vi "Stanford Research 830 Expand Offset and Output Channel.vi"() -> ()   [LabVIEW 2019]
doc: "This example shows how to configure all the channel-related parameters of the instrument to get the desired output value."
uses:
  Stanford Research 830.lvlib
panel:
  in  "Offset/Expand Parameter (1: X)":u16(ring)=1 items=["X"=1, "Y"=2, "R"=3]
  in  "Expand (0: x1)":u16(ring) items=["x1", "x10", "x100"]
  in  "Channel 1 Display With Ratio (0: None)":u16(ring) items=["None", "Aux In 1", "Aux In 2"]
  in  "Channel 1 Display (0: X)":u16(ring) items=["X", "R", "X Noise", "Aux In 1", "Aux In 2"]
  in  "Manual Offset (40)":dbl=40.0
  in  "Auto Offset (F: Disable)":bool
  in  "VISA resource name":refnum<visa-resource-name>
  # "(c) 2006 National Instruments.  ALL RIGHTS RESERVED."
  # "Offset/Expand Configuration"
  # "Channel Display Configuration"
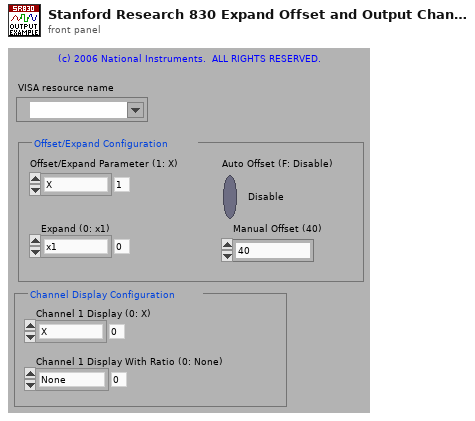
[diagram p1: front panel]
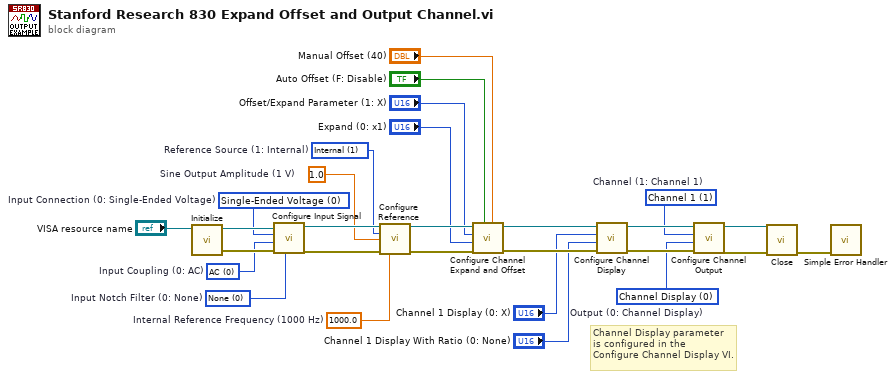
[diagram p0: block diagram]
diagram:
  w3 = u16 0 items=["Channel Display", "X or Y"]  # Output (0: Channel Display)
  w4 = u16 1 items=["Channel 1"=1, "Channel 2"=2]  # Channel (1: Channel 1)
  w11 = u16 0 items=["Single-Ended Voltage", "Differential Voltage", "1 MOhm Current Gain", "100 MOhm Current Gain"]  # Input Connection (0: Single-Ended Voltage)
  w12 = u16 0 items=["None", "Line Notch", "2x Line Notch", "Both Notch Filters"]  # Input Notch Filter (0: None)
  w13 = u16 0 items=["AC", "DC"]  # Input Coupling (0: AC)
  w14 = 1.0  # Sine Output Amplitude (1 V)
  w15 = 1000.0  # Internal Reference Frequency (1000 Hz)
  w16 = u16 1 items=["External", "Internal"]  # Reference Source (1: Internal)
  # "Channel Display parameter is configured in the Configure Channel Display VI."
  n1 = call "Initialize.vi"("VISA resource name"="VISA resource name") -> ("error out"=w26:errorcluster, "VISA resource name out"=w27:refnum<visa-resource-name>)  [unwired: 9 in]
  n2 = call "Configure Input Signal.vi"("Input Notch Filter (0: None)"=w12, "error in (no error)"=w26, "Input Coupling (0: AC)"=w13, "Input Connection (0: Single-Ended Voltage)"=w11, "VISA resource name"=w27) -> ("error out"=w23:errorcluster, "VISA resource name out"=w24:refnum<visa-resource-name>)  [unwired: 5 in]
  n3 = call "Configure Reference.vi"("VISA resource name"=w24, "Reference Source (1: Internal)"=w16, "Sine Output Amplitude (1 V)"=w14, "error in (no error)"=w23, "Internal Reference Frequency (1000 Hz)"=w15) -> ("VISA resource name out"=w21:refnum<visa-resource-name>, "error out"=w22:errorcluster)  [unwired: 9 in]
  n4 = call "Configure Channel Expand and Offset.vi"("Manual Offset (0)"="Manual Offset (40)", "Auto Offset (F: Disable)"="Auto Offset (F: Disable)", "error in (no error)"=w22, "Expand (0: x1)"="Expand (0: x1)", "Offset/Expand Parameter (1: X)"="Offset/Expand Parameter (1: X)", "VISA resource name"=w21) -> ("error out"=w9:errorcluster, "VISA resource name out"=w10:refnum<visa-resource-name>)  [unwired: 4 in]
  n5 = call "Configure Channel Display.vi"("error in (no error)"=w9, "Channel 1 Display With Ratio (0: None)"="Channel 1 Display With Ratio (0: None)", "Channel 1 Display (0: X)"="Channel 1 Display (0: X)", "VISA resource name"=w10) -> ("error out"=w7:errorcluster, "VISA resource name out"=w8:refnum<visa-resource-name>)  [unwired: 6 in]
  n6 = call "Configure Channel Output.vi"("error in (no error)"=w7, "Output (0: Channel Display)"=w3, "Channel (1: Channel 1)"=w4, "VISA resource name"=w8) -> ("error out"=w19:errorcluster, "VISA resource name out"=w20:refnum<visa-resource-name>)  [unwired: 6 in]
  n7 = call "Close.vi"("error in (no error)"=w19, "VISA resource name"=w20) -> ("error out"=w25:errorcluster)  [unwired: 9 in]
  n8 = call <vilib>:"Simple Error Handler.vi"("error in (no error)"=w25) -> ()  [unwired: 4 in, 5 out]
